vi "Maxi Gauge-RW Filter time.vi"(0 "VISA-Ressource in":refnum<visa-resource-name>, 1 "Sensor 1 Set":i8(ring)=1 items=["fast", "standard", "slow"], 2 "Sensor 2 Set":i8(ring)=1 items=["fast", "standard", "slow"], 3 "Sensor 3 Set":i8(ring)=1 items=["fast", "standard", "slow"], 4 "Sensor 4 Set":i8(ring)=1 items=["fast", "standard", "slow"], 5 "Fehler (Eingang)":errorcluster, 6 "Node address":i8=-1 min=-1 max=31 step=1, 7 "Sensor 5 Set":i8(ring)=1 items=["fast", "standard", "slow"], 8 "W/R":bool, 9 "Sensor 6 Set":i8(ring)=1 items=["fast", "standard", "slow"]) -> (12 "Sensor 1 Get":i8(ring)=2 items=["fast", "standard", "slow"], 13 "Sensor 6 Get":i8(ring)=2 items=["fast", "standard", "slow"], 14 "VISA-Ressource out":refnum<visa-resource-name>, 15 "Sensor 2 Get":i8(ring)=2 items=["fast", "standard", "slow"], 16 "Sensor 3 Get":i8(ring)=2 items=["fast", "standard", "slow"], 17 "Sensor 4 Get":i8(ring)=2 items=["fast", "standard", "slow"], 18 "Sensor 5 Get":i8(ring)=2 items=["fast", "standard", "slow"], 19 "Fehler (Ausgang)":errorcluster)   [LabVIEW 2013, in "Maxi Gauge.lvlib"]
uses:
  <instrlib>/Maxi Gauge/Maxi Gauge.lvlib
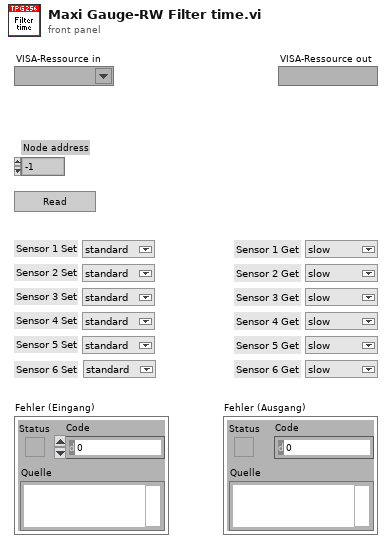
[diagram p1: front panel]
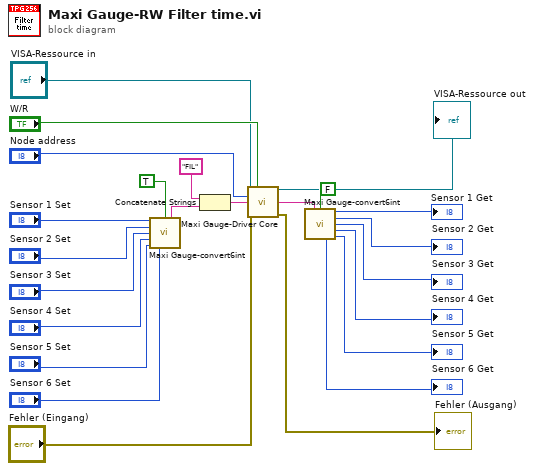
[diagram p0: block diagram]
diagram:
  n1 = call <instrlib>:"Maxi Gauge-convert6int.vi"("Integer1 in"="Sensor 1 Set", "W/R [W: Int in; Str out ]"=TRUE, "Integer2 in"="Sensor 2 Set", "Integer3 in"="Sensor 3 Set", "Integer4 in"="Sensor 4 Set", "Integer5 in"="Sensor 5 Set", "Integer6 in"="Sensor 6 Set") -> ("String out"=w8:string)  [unwired: 2 in, 6 out]
  n2 = Concatenate Strings("FIL", w8) -> (w5:string)
  n3 = call <instrlib>:"Maxi Gauge-Driver Core.vi"("VISA-Ressource in"="VISA-Ressource in", "Write/Read"="W/R", "Node address"="Node address", "Command"=w5, "Fehler (Eingang)"="Fehler (Eingang)") -> ("VISA-Ressource out"=→"VISA-Ressource out":refnum<visa-resource-name>, "String Out"=w6:string, "Fehler (Ausgang)"=→"Fehler (Ausgang)":errorcluster)  [unwired: 8 in]
  n4 = call <instrlib>:"Maxi Gauge-convert6int.vi"("String in"=w6, "W/R [W: Int in; Str out ]"=FALSE) -> ("Integer1 out"=→"Sensor 1 Get":u8, "Integer2 out"=→"Sensor 2 Get":u8, "Integer3 out"=→"Sensor 3 Get":u8, "Integer4 out"=→"Sensor 4 Get":u8, "Integer6 out"=→"Sensor 6 Get":u8, "Integer5 out"=→"Sensor 5 Get":u8)  [unwired: 7 in, 1 out]
